vi "TalonFXSetters.vi"   [LabVIEW 2023]
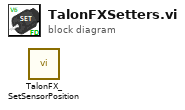
[diagram p0: block diagram]
diagram:
  n1 = call <vilib>:"TalonFX_SetSensorPosition.vi"() -> ()  [unwired: 12 in]
